vi "GUI_Pico.vi"() -> ()   [LabVIEW 2013]
uses:
  Shared/GUI_Template/GUI_master/tcp_new_data_event.ctl
  Shared/GUI_Template/GUI_master/tcp new data cluster.ctl
panel:
  in  "RelativeSettings.Axis 2.StepSize::1":dbl=29.9701 caption="Axis 2 StepSize" min=0.0 max=500.0 format="%_4p"
  in  "RelativeSettings.Axis 2.Position::1":dbl=29.9701 caption="Axis 2 Position" min=0.0 max=0.0 format="%_4p"
  in  "RelativeSettings.Axis 1.StepSize::1":dbl=29.9701 caption="Axis 1 Stepsize" min=0.0 max=500.0 format="%_4p"
  in  "RelativeSettings.Axis 1.Position::1":dbl=29.9701 caption="Axis 1 Position" min=0.0 max=0.0 format="%_4p"
  in  "RelativeMove.Axis 2.CW::1":bool
  in  "RelativeMove.Axis 2.CCW::1":bool caption="RelativeMove.Axis. 2.CCW::1"
  in  "RelativeMove.Axis 1.CW::1":bool
  in  "RelativeMove.Axis 1.CCW::1":bool
  in  "ActiveMotorName::1":string
  in  "ActiveMotor":u16(ring) items=["M21-amp1Out", "DogLeg"]
  in  "GUIdevice 1":string="LB-Picopad1"
  out "Names":string[](array[string])
  in  "insert tag":bool=TRUE
  in  "stop":bool
  out "tcp data event":T1
  out "error IO 2":errorcluster
  # "LB-Picopad1"
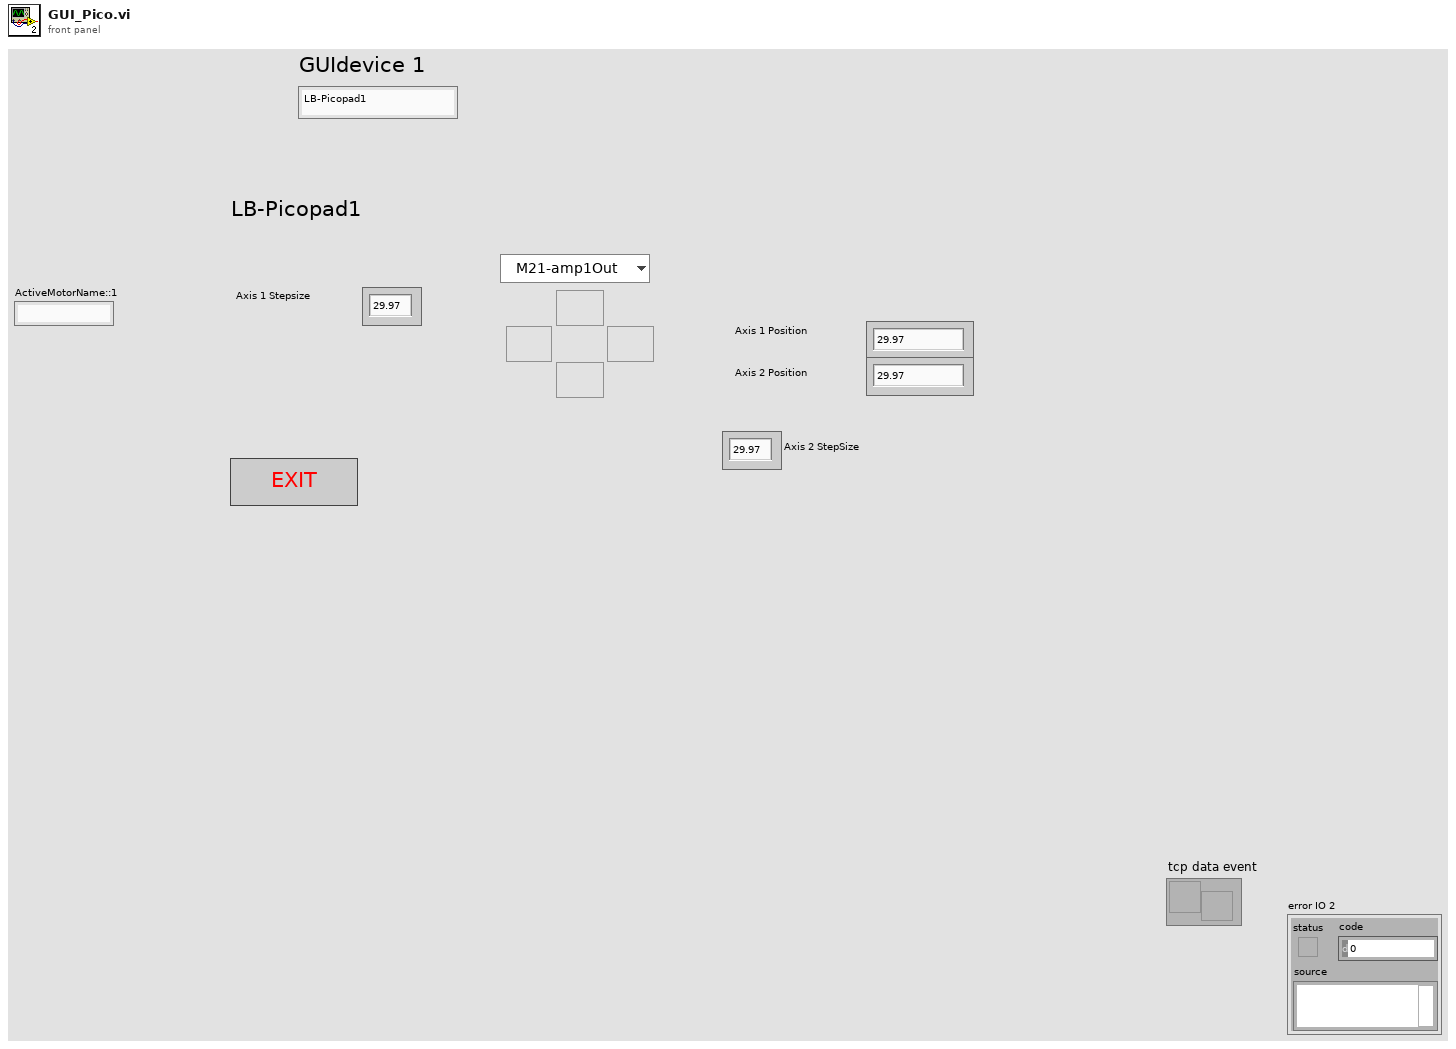
[diagram p1: front panel]
types:
  T1 = typedef "tcp_new_data_event.ctl" = refnum<user-event>
  T2 = typedef "tcp new data cluster.ctl" = cluster{"EventEnum":enum16{"new data", "connection status update"}, "Device name":string}
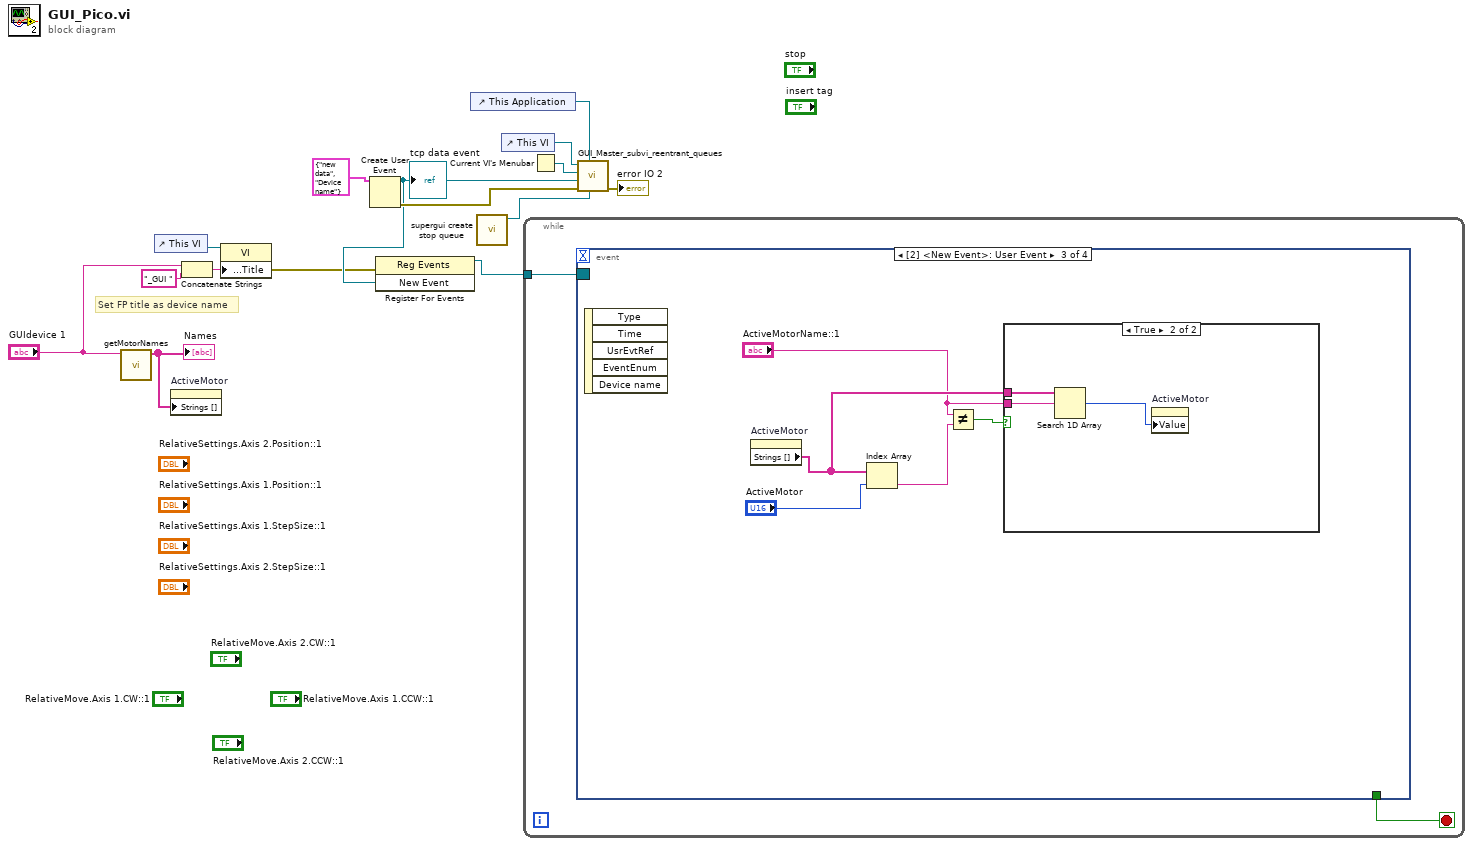
[diagram p0: block diagram]
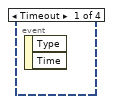
[diagram p2: hidden frame]
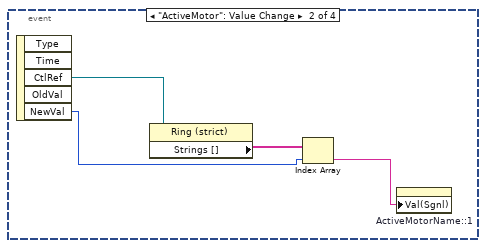
[diagram p3: hidden frame]
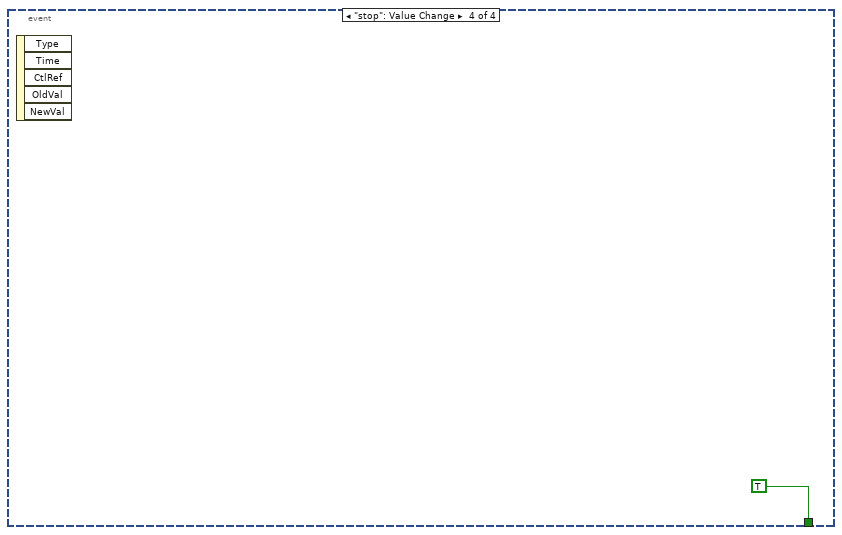
[diagram p5: hidden frame]
diagram:
  # "Set FP title as device name"
  n1 = call "getMotorNames.vi"("DeviceName"="GUIdevice 1") -> ("elements"=w7:string[])  [unwired: 10 in]
  "Names" <- w7
  n2 = control-ref of="This VI"() -> (w4:refnum<vi>)
  n3 = property on="ActiveMotor" class="Ring (strict)"("Strings []"=w7) -> ()  [unwired: 2 in, 2 out]
  n4 = Concatenate Strings("GUIdevice 1", "_GUI ") -> (w3:string)
  n5 = property class="VI"(reference=w4, "Front Panel.Title"=w3) -> (error out=w1:errorcluster)  [unwired: 1 in, 1 out]
  n6 = Create User Event(user event datatype=T2 {"EventEnum"=enum."new data", "Device name"="Device name"} ("New Event")) -> (user event=w9:refnum<user-event>, error out=w11:errorcluster)  [unwired: 1 in]
  "tcp data event" <- w9
  n7 = register-events(error in=w1, w9) -> (reference out=w8:refnum<event-registration>)  [unwired: 1 in, 1 out]
  n8 = control-ref of="This Application"() -> (w10:refnum<vi>)
  n9 = call "supergui create stop queue.vi"() -> ("STOP Queue out"=w6:refnum<queue>)  [unwired: 11 in]
  n10 = control-ref of="This VI"() -> (w14:refnum<vi>)
  n11 = while {
    tunnel: w8 -> [w16]
    stop <- w17 stop-if-true
    n12 = event shown="[2] <New Event>: User Event" {
      selector: w16 -> [_ _ _ _]
      dyn-events: _ -> [_ _ _ _]
      timeout: _ -> [_ _ _ _]
      tunnel: [_ _ _ TRUE] -> w17
      event Timeout {
        n13 = event-data() -> ()  [unwired: 1 in, 2 out]
      }
      event "ActiveMotor": Value Change {
        n14 = event-data() -> ("CtlRef"=w21:refnum<vi>, "NewVal"=w19:u16)  [unwired: 1 in, 3 out]
        n15 = property class="Ring (strict)"(reference=w21) -> ("Strings []"=w20:string[])  [unwired: 1 in, 2 out]
        n16 = Index Array(array=w20, index=w19) -> (element=w18:string)
        n17 = property on="ActiveMotorName::1" class="Str"("Val(Sgnl)"=w18) -> ()  [unwired: 2 in, 2 out]
      }
      event User Event {
        n18 = event-data() -> ()  [unwired: 1 in, 5 out]
        n19 = property on="ActiveMotor" class="Ring (strict)"() -> ("Strings []"=w23:string[])  [unwired: 2 in, 2 out]
        n20 = Index Array(array=w23, index="ActiveMotor") -> (element=w25:string)
        n21 = Not Equal?(x="ActiveMotorName::1", y=w25) -> (x != y?=w24:bool)
        n22 = case shown="True" w24 {
          tunnel: w23 -> [_ w29]
          tunnel: "ActiveMotorName::1" -> [_ w28]
          frame False {
          }
          frame True {
            n23 = Search 1D Array(1D array=w29, element=w28) -> (index of element=w27:i32)  [unwired: 1 in]
            n24 = property on="ActiveMotor" class="Ring (strict)"("Value"=w27) -> ()  [unwired: 2 in, 2 out]
          }
        }
      }
      event "stop": Value Change {
        n25 = event-data() -> ()  [unwired: 1 in, 5 out]
      }
    }
  }
  n26 = Current VI's Menubar() -> (w13:refnum<k9>)
  n27 = call "GUI_Master_subvi_reentrant_queues.vi"("STOP Queue in"=w6, "This Application"=w10, "error in (no error)"=w11, "tcp data event"=w9, "Caller menu reference"=w13, "Caller VI ref"=w14) -> ("error out"=→"error IO 2":errorcluster)  [unwired: 5 in]
